vi "3-8.vi"() -> ()   [LabVIEW 2014]
panel:
  out "?":string
  out "Warning?":bool
  in  "Min Temp.":dbl
  in  "Max Temp.":dbl
  in  "Current Temp.":dbl
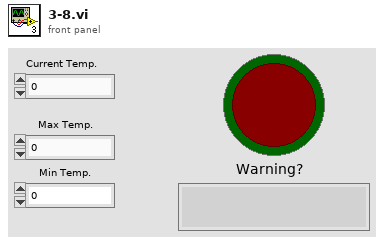
[diagram p1: front panel]
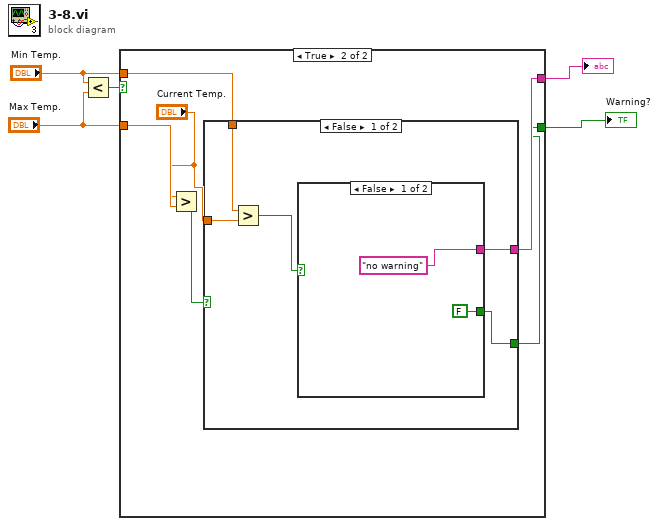
[diagram p0: block diagram]
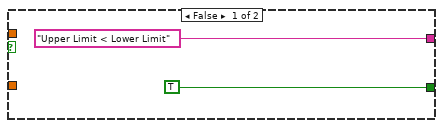
[diagram p2: hidden frame]
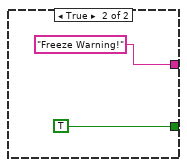
[diagram p3: hidden frame]
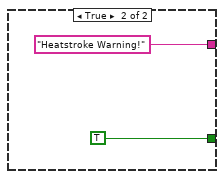
[diagram p4: hidden frame]
diagram:
  n1 = Less?(x="Min Temp.", y="Max Temp.") -> (x < y?=w3:bool)
  n2 = case shown="True" w3 {
    tunnel: [TRUE w10] -> w5
    tunnel: ["Upper Limit < Lower Limit" w11] -> w4
    tunnel: "Max Temp." -> [_ w13]
    tunnel: "Min Temp." -> [_ w9]
    frame False {
    }
    frame True {
      n3 = Greater?(x="Current Temp.", y=w13) -> (0:w12:bool)
      n4 = case shown="False" w12 {
        tunnel: [w14 "Heatstroke Warning!"] -> w11
        tunnel: [w15 TRUE] -> w10
        tunnel: w9 -> [w18 _]
        tunnel: "Current Temp." -> [w17 _]
        frame False {
          n5 = Greater?(x=w18, y=w17) -> (0:w16:bool)
          n6 = case shown="False" w16 {
            tunnel: [FALSE TRUE] -> w15
            tunnel: ["no warning" "Freeze Warning!"] -> w14
            frame False {
            }
            frame True {
            }
          }
        }
        frame True {
        }
      }
    }
  }
  "Warning?" <- w5
  "?" <- w4
